vi "Create_Deadband.vi"(3 "Input":dbl) -> (0 "Output":dbl, 1 "Not Zero?":bool)   [LabVIEW 2019]
uses:
  Globals/Sensor_Values.vi
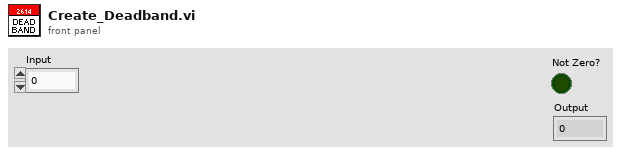
[diagram p1: front panel]
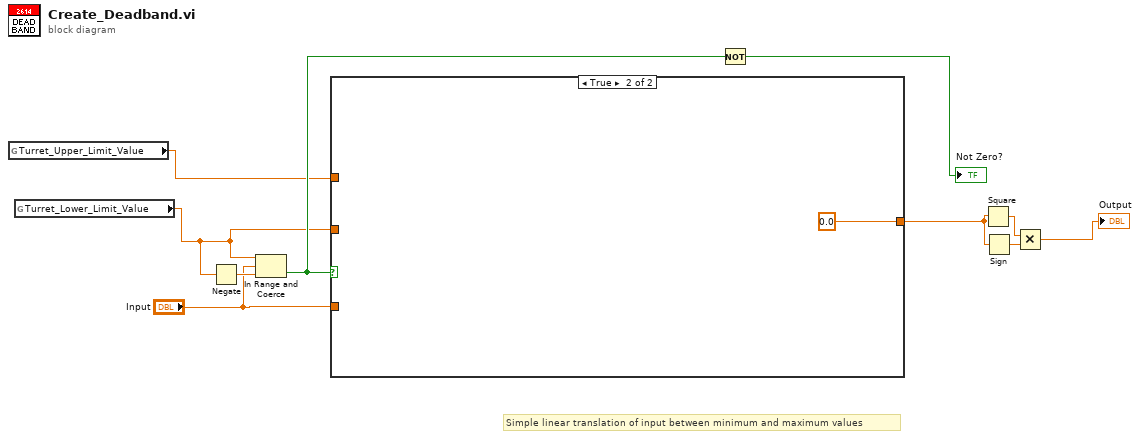
[diagram p0: block diagram]
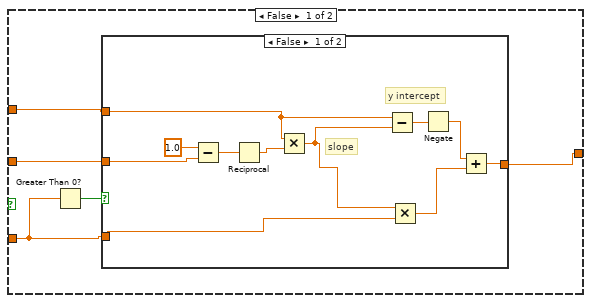
[diagram p2: hidden frame]
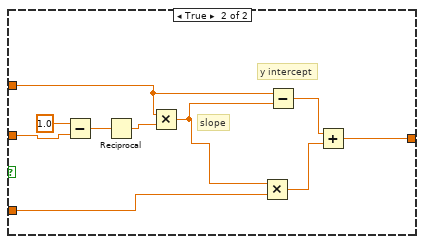
[diagram p3: hidden frame]
diagram:
  # "Simple linear translation of input between minimum and maximum values"
  n1 = global read "Sensor_Values.vi" "Turret_Upper_Limit_Value"() -> (w2:dbl)
  n2 = global read "Sensor_Values.vi" "Turret_Lower_Limit_Value"() -> (w1:dbl)
  n3 = Negate(x=w1) -> (-x=w10:dbl)
  n4 = In Range and Coerce(upper limit=w1, x="Input", lower limit=w10) -> (In Range?=w8:bool)  [unwired: 1 out]
  n5 = case shown="True" w8 {
    tunnel: w1 -> [w14 _]
    tunnel: "Input" -> [w11 _]
    tunnel: [w13 0.0 ("Output")] -> w4
    tunnel: w2 -> [w15 _]
    frame False {
      n6 = Greater Than 0?(x=w11) -> (x > 0?=w12:bool)
      n7 = case shown="False" w12 {
        tunnel: w15 -> [w21 w33]
        tunnel: w14 -> [w22 w32]
        tunnel: w11 -> [w20 w31]
        tunnel: [w19 w28] -> w13
        frame False {
          # "y intercept"
          # "slope"
          n8 = Subtract(x=1.0, y=w22) -> (x-y=w24:dbl)
          n9 = Reciprocal(x=w24) -> (1/x=w25:dbl)
          n10 = Multiply(x=w21, y=w25) -> (x*y=w16:dbl)
          n11 = Subtract(x=w21, y=w16) -> (x-y=w18:dbl)
          n12 = Multiply(x=w16, y=w20) -> (x*y=w26:dbl)
          n13 = Negate(x=w18) -> (-x=w17:dbl)
          n14 = Add(x=w17, y=w26) -> (x+y=w19:dbl)
        }
        frame True {
          # "y intercept"
          # "slope"
          n15 = Subtract(x=1.0, y=w32) -> (x-y=w35:dbl)
          n16 = Reciprocal(x=w35) -> (1/x=w34:dbl)
          n17 = Multiply(x=w33, y=w34) -> (x*y=w27:dbl)
          n18 = Multiply(x=w27, y=w31) -> (x*y=w30:dbl)
          n19 = Subtract(x=w33, y=w27) -> (x-y=w29:dbl)
          n20 = Add(x=w29, y=w30) -> (x+y=w28:dbl)
        }
      }
    }
    frame True {
    }
  }
  n21 = Not(x=w8) -> (.not. x?=→"Not Zero?":bool)
  n22 = Square(x=w4) -> (x^2=w6:dbl)
  n23 = Sign(1:w4) -> (0:w5:dbl)
  n24 = Multiply(x=w6, y=w5) -> (x*y=→"Output":dbl)
